vi "Element Height.vi"() -> (3 "Element Height":i16)   [LabVIEW 2020, in "Value Editor Template.lvclass"]
uses:
  Value Editor Template.lvclass/Value Editor Template.ctl
  Value Editor Template.lvclass
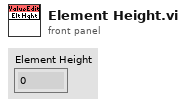
[diagram p1: front panel]
types:
  T1 = typedef "LVRectTypeDef.ctl" = cluster{"Left":i16, "Top":i16, "Right":i16, "Bottom":i16}
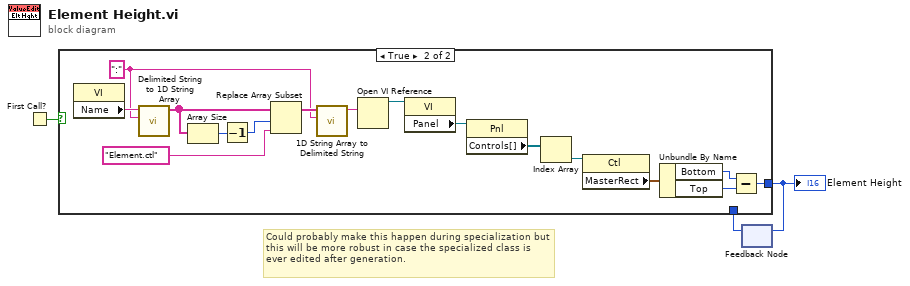
[diagram p0: block diagram]
diagram:
  # "Could probably make this happen during specialization but this will be more robust in case the specialized class is ever edited after generation."
  n1 = First Call?() -> (First Call?: T/F=w3:bool)
  n2 = feedback #1() -> (w1:i16)  [unwired: 1 in]
  n3 = case shown="True" w3 {
    tunnel: [w4 w5] -> w2
    tunnel: w1 -> [w4 _]
    frame False {
    }
    frame True {
      w14 = ":" ("delimiter")
      n4 = property class="VI"() -> ("Name"=w20:string)  [unwired: 2 in, 2 out]
      n5 = call <vilib>:"Delimited String to 1D String Array.vi"("delimiter"=w14, "delimited string"=w20) -> ("string array"=w19:string[])  [unwired: 9 in]
      n6 = Array Size(array=w19) -> (size(s)=w18:i32)
      n7 = Decrement(x=w18) -> (x-1=w17:i32)
      n8 = Replace Array Subset(array=w19, new element="Element.ctl", index=w17) -> (w15:string[])
      n9 = call <vilib>:"1D String Array to Delimited String.vi"("delimiter"=w14, "string array"=w15) -> ("delimited string"=w13:string)  [unwired: 9 in]
      n10 = Open VI Reference(vi path=w13) -> (vi reference=w12:refnum<vi>)  [unwired: 5 in, 1 out]
      n11 = property class="VI"(reference=w12) -> ("Panel"=w11:refnum<vi>)  [unwired: 1 in, 2 out]
      n12 = property class="Pnl"(reference=w11) -> ("Controls[]"=w10:refnum<vi>[])  [unwired: 1 in, 2 out]
      n13 = Index Array(array=w10) -> (element=w9:refnum<vi>)  [unwired: 1 in]
      n14 = property class="Ctl"(reference=w9) -> ("MasterRect"=w8:T1)  [unwired: 1 in, 2 out]
      n15 = Unbundle By Name(w8) -> ("Bottom"=w7:i16, "Top"=w6:i16)
      n16 = Subtract(x=w7, y=w6) -> (x-y=w5:i16)
    }
  }
  "Element Height" <- w2
  n17 = feedback-in #1(w2) -> ()
